vi "BumplessTransfer_Execute.vi"(4 "Rate 2":dbl, 6 "Rate 1":dbl, 8 "Time":dbl=-1.0, 9 "Select 2":bool, 10 "Input 2":dbl, 11 "Input 1":dbl) -> (3 "Output":dbl)   [LabVIEW 2019, in "Trajectory_Library.lvlib"]
doc: "This VI averages the last seven samples of an analog value. The sample rate is determined by how often this VI is called."
uses:
  Trajectory_Library.lvlib
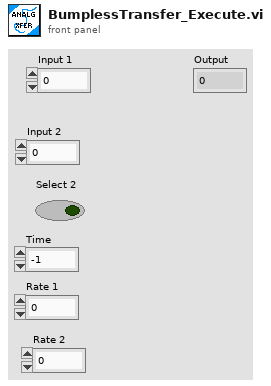
[diagram p1: front panel]
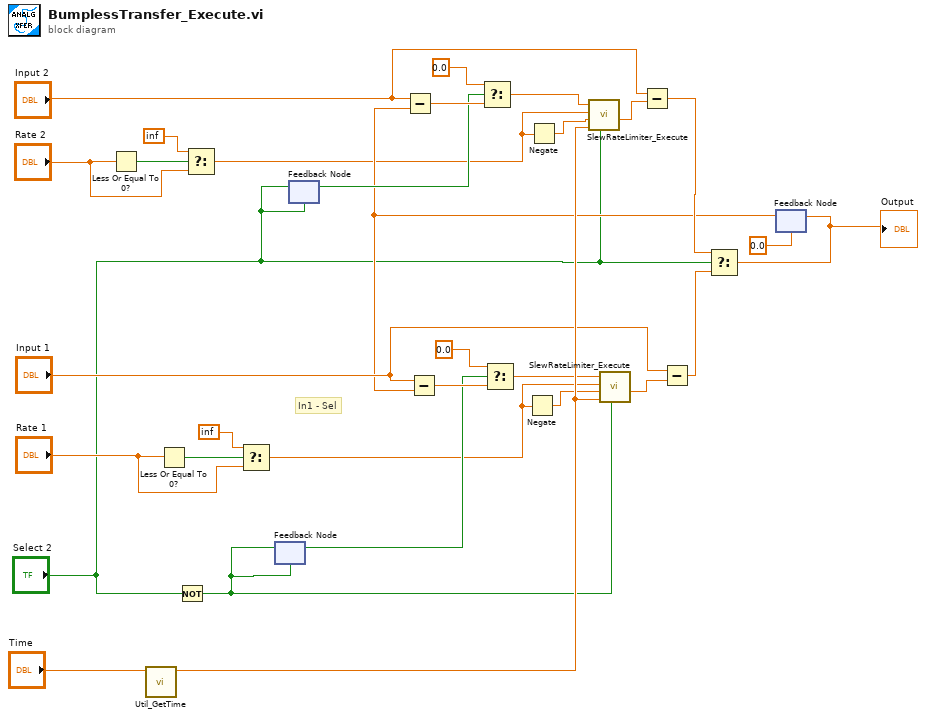
[diagram p0: block diagram]
diagram:
  # "In1 - Sel"
  n1 = Less Or Equal To 0?(x="Rate 2") -> (x <= 0?=w27:bool)
  n2 = call "Util_GetTime.vi"("Pass_Through_Time"="Time") -> ("FPGA_Time_Seconds"=w24:dbl)  [unwired: 9 in, 1 out]
  n3 = Less Or Equal To 0?(x="Rate 1") -> (x <= 0?=w30:bool)
  n4 = Not(x="Select 2") -> (.not. x?=w3:bool)
  n5 = Select(t=inf, s=w27, f="Rate 2") -> (s? t:f=w5:dbl)
  n6 = Select(t=inf, s=w30, f="Rate 1") -> (s? t:f=w2:dbl)
  n7 = feedback #1(w3) -> (w16:bool)
  n8 = feedback-in #1(w3) -> ()
  n9 = feedback-in #2("Select 2") -> ()
  n10 = feedback #2("Select 2") -> (w20:bool)
  n11 = Negate(x=w2) -> (-x=w1:dbl)
  n12 = Negate(x=w5) -> (-x=w4:dbl)
  n13 = feedback #3(0.0) -> (w9:dbl)
  n14 = Subtract(x="Input 2", y=w9) -> (x-y=w23:dbl)
  n15 = Subtract(x="Input 1", y=w9) -> (x-y=w18:dbl)
  n16 = Select(t=0.0, s=w20, f=w23) -> (s? t:f=w22:dbl)
  n17 = Select(t=0.0, s=w16, f=w18) -> (s? t:f=w17:dbl)
  n18 = call "SlewRateLimiter_Execute.vi"("Enable"="Select 2", "Time"=w24, "NegativeRate"=w4, "PositiveRate"=w5, "Input"=w22) -> ("Output"=w7:dbl)  [unwired: 5 in, 1 out]
  n19 = call "SlewRateLimiter_Execute.vi"("Enable"=w3, "Time"=w24, "NegativeRate"=w1, "PositiveRate"=w2, "Input"=w17) -> ("Output"=w14:dbl)  [unwired: 5 in, 1 out]
  n20 = Subtract(x="Input 2", y=w7) -> (x-y=w10:dbl)
  n21 = Subtract(x="Input 1", y=w14) -> (x-y=w12:dbl)
  n22 = Select(t=w10, s="Select 2", f=w12) -> (s? t:f=w11:dbl)
  "Output" <- w11
  n23 = feedback-in #3(w11) -> ()
